vi "All_Multiplexer_Ch_Numbers.vi"(0 "Channel Numbers":i16[](array[numeric])) -> (1 "Multiplexer Ch No":i16[](array[numeric]), 2 "ADC Ch No":i16[](array[numeric]))   [LabVIEW 2012]
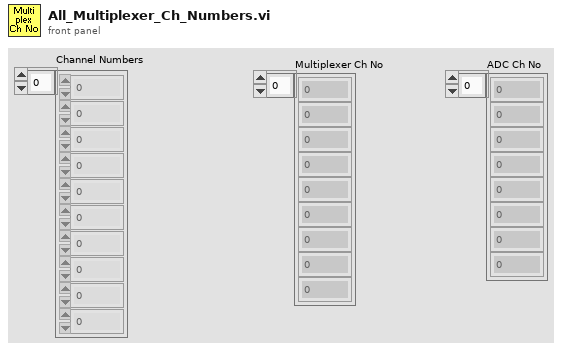
[diagram p1: front panel]
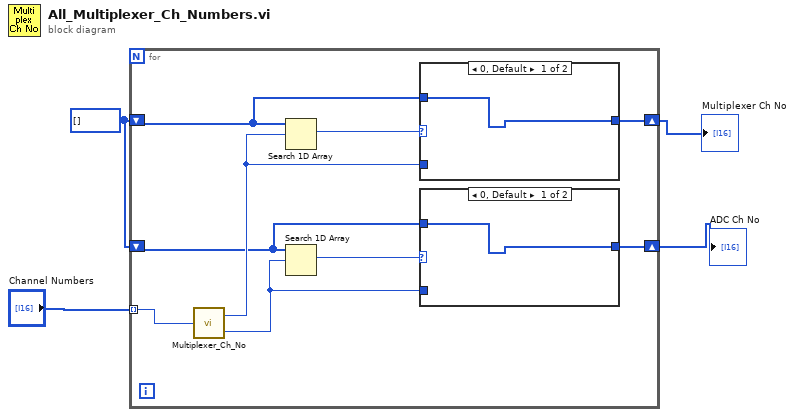
[diagram p0: block diagram]
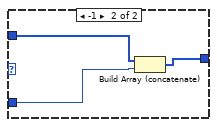
[diagram p2: hidden frame]
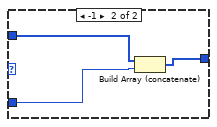
[diagram p3: hidden frame]
diagram:
  w3 = i16[] []
  n1 = for {
    tunnel: "Channel Numbers" -> [w13] mode=indexing
    shift-right: [w9] -> w1
    shift-left: w3 -> [w11]
    shift-right: [w8] -> w2
    shift-left: w3 -> [w7]
    n2 = call "Multiplexer_Ch_No.vi"("Channel Number"=w13) -> ("Multiplexer Ch No"=w10:i16, "ADC Ch No"=w5:i16)
    n3 = Search 1D Array(1D array=w11, element=w10) -> (index of element=w12:i32)  [unwired: 1 in]
    n4 = Search 1D Array(1D array=w7, element=w5) -> (index of element=w6:i32)  [unwired: 1 in]
    n5 = case shown="0, Default" w12 {
      tunnel: w11 -> [w18 w21]
      tunnel: w10 -> [_ w20]
      tunnel: [w18 w19] -> w9
      frame 0, Default {
      }
      frame -1 {
        n6 = Build Array (concatenate)(w21, w20) -> (w19:i16[])
      }
    }
    n7 = case shown="0, Default" w6 {
      tunnel: w7 -> [w14 w17]
      tunnel: w5 -> [_ w16]
      tunnel: [w14 w15] -> w8
      frame 0, Default {
      }
      frame -1 {
        n8 = Build Array (concatenate)(w17, w16) -> (w15:i16[])
      }
    }
  }
  "ADC Ch No" <- w2
  "Multiplexer Ch No" <- w1
